vi "Insert book exchange into jos_modules_menu.vi"(1 "menuid":string, 4 "moduleid":string) -> ()   [LabVIEW 2010]
doc: "This example opens a connection to a database specified by the Connection string (replace the DNS name with your database) inserts a new row into the table \"myOtherTable\" (replace the SQL string with your own SQL query)."
panel:
  out "concatenated string":string
  out "error out":errorcluster
  in  "Command Text":string="INSERT INTO jos_menu\n (id, menutype, name, alias, link to article, type, published, parent, componentid, sublevel, browserNav, access, utaccess, params, lft, rgt, home)\nVALUES ('id', 'unpublished', 'name', 'alias', 'index.php?option=com_content&view=article&id=117', 'component', '1', '0', '20', '0', '0', '0', '0', 'show_noauth=\nshow_title=\nlink_titles=\nshow_intro=\nshow_section=\nlink_section=\nshow_category=\nlink_category=\nshow_author=\nshow_create_date=\nshow_modify_date=\nshow_item_navigation=\nshow_readmore=\nshow_vote=\nshow_icons=\nshow_pdf_icon=\nshow_print_icon=\nshow_email_icon=\nshow_hits=\nfeed_summary=\npage_title=\nshow_page_title=1\npageclass_sfx=\nmenu_image=-1\nsecure=0\n', '0', '0', '0');"
  in  "ConnectionString":string="DSN=stusbooks;"
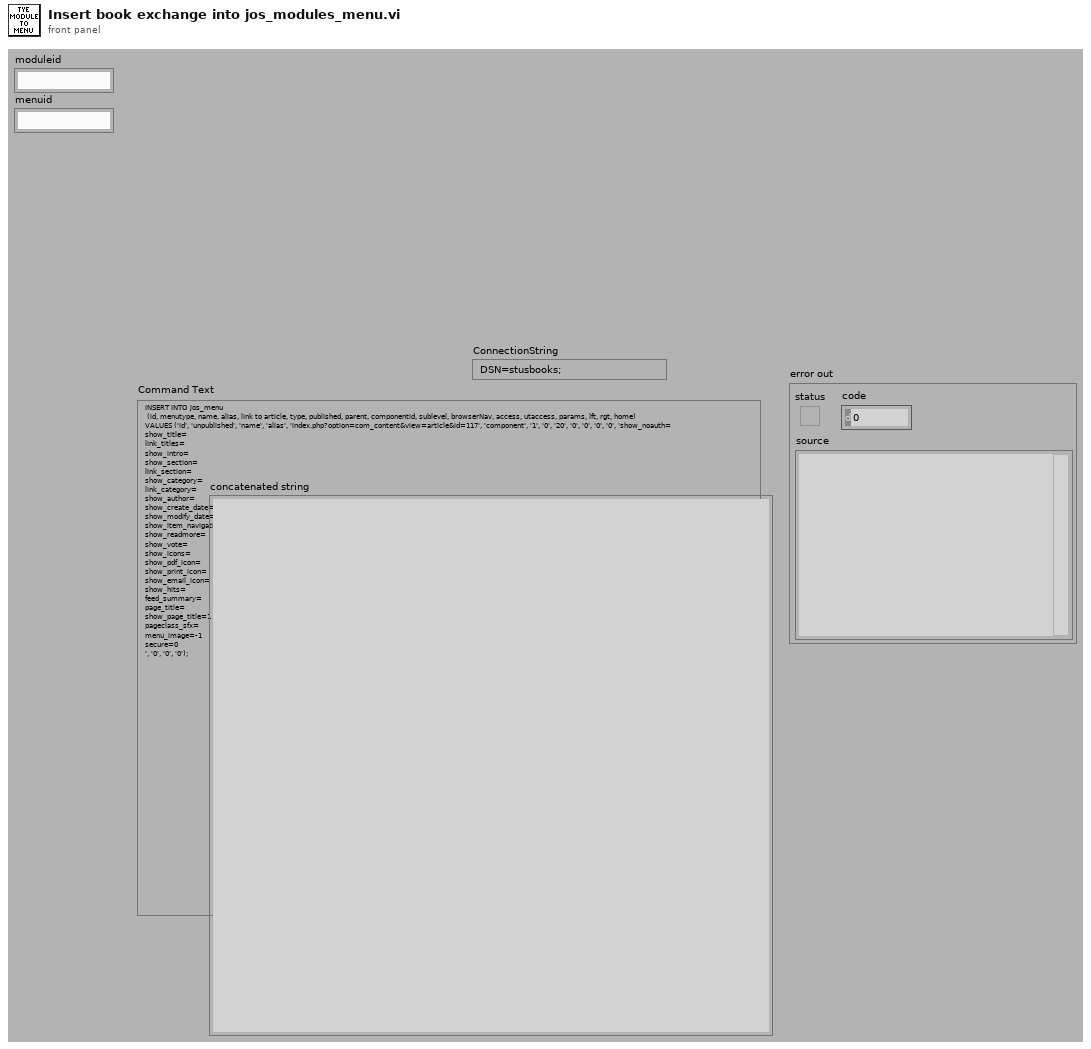
[diagram p1: front panel]
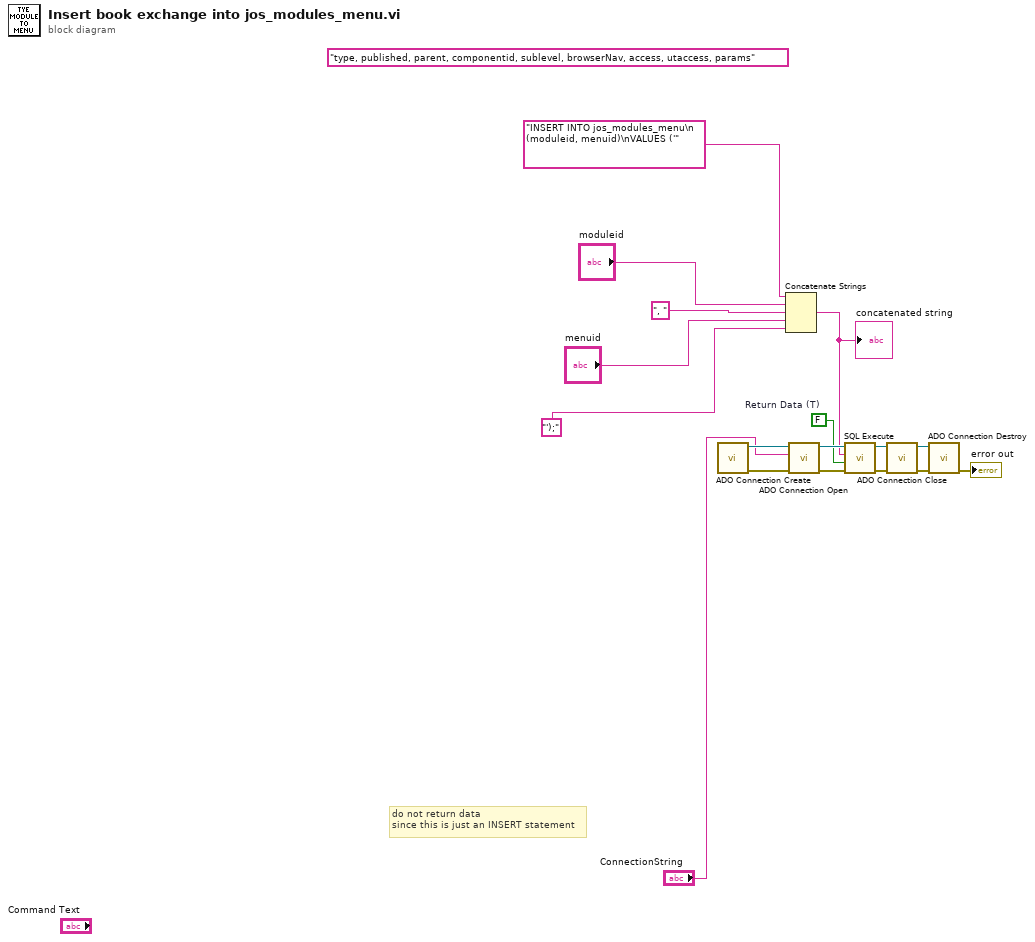
[diagram p0: block diagram]
diagram:
  (unwired) "type, published, parent, componentid, sublevel, browserNav, access, utaccess, params"
  w7 = FALSE  # Return Data (T)
  # "do not return data\nsince this is just an INSERT statement"
  n1 = call "ADO Connection Create.vi"() -> ("error out"=w16:errorcluster, "ADODB._Connection Out"=w17:refnum<k7>)  [unwired: 10 in]
  n2 = Concatenate Strings("INSERT INTO jos_modules_menu\n (moduleid, menuid)\nVALUES ('", "moduleid", ", " ("string"), "menuid", "');" ("string")) -> (w6:string)
  "concatenated string" <- w6
  n3 = call "ADO Connection Open.vi"("error in (no error)"=w16, "ConnectionString"="ConnectionString", "ADODB._Connection In"=w17) -> ("error out"=w13:errorcluster, "ADODB._Connection Out"=w14:refnum<k7>)  [unwired: 7 in]
  n4 = call "SQL Execute.vi"("error in (no error)"=w13, "Return Data (T)"=w7, "Command Text"=w6, "ADODB._Connection In"=w14) -> ("error out"=w12:errorcluster, "ADODB._Connection Out"=w11:refnum<k7>)  [unwired: 4 in, 2 out]
  n5 = call "ADO Connection Close.vi"("error in (no error)"=w12, "ADODB._Connection In"=w11) -> ("error out"=w10:errorcluster, "ADODB._Connection Out"=w9:refnum<k7>)  [unwired: 8 in]
  n6 = call "ADO Connection Destroy.vi"("error in (no error)"=w10, "ADODB._Connection In"=w9) -> ("error out"=→"error out":errorcluster)  [unwired: 9 in]
